vi "RT Driver VI.vi"(7 "Operation":T1, 11 "Device Reference in":T2 format="%.0x") -> (0 "Error Code":i32)   [LabVIEW 2019, in "Control Addon Engine.lvlib"]
uses:
  Control Addon Engine.lvlib
  <vilib>/NI VeriStand/Custom Device API/Custom Device Item Ref.ctl
  <vilib>/NI VeriStand/Custom Device API/Model Interface Driver VI Operation.ctl
  Types/RT Driver State Variables.ctl
  Types/RT Configuration.ctl
  Addon Shared/Types/Gain Schedule.ctl
  Addon Shared/Types/Compiled Settings.ctl
  Addon Shared/Types/Compiled PID Settings.ctl
  <vilib>/NI VeriStand/Custom Device API/Block Data Reference.ctl
  <vilib>/NI VeriStand/Custom Device API/Data Reference.ctl
  Addon Shared/Types/Compiled Industrial Settings.ctl
  Addon Shared/Types/Compiled Industrial Parameters.ctl
  <vilib>/NI/NIVS Inline Async API/_VS Inline Async API/VS Inline Async API/VS Inline Async API.lvclass
  <vilib>/NI/NIVS Inline Async API/_VS Inline Async API/VS Inline Async API/Types/Error Handling Settings.ctl
  <vilib>/NI VeriStand/Custom Device API/NI VeriStand - Get Channel Values by Block Data Reference.vi
  <vilib>/addons/control/pid/pid.llb/PID Advanced (DBL Array).vi
  <vilib>/NI VeriStand/Custom Device API/NI VeriStand - Set Channel Values by Block Data Reference.vi
  SubVIs/Get PID Gains from Schedule.vi
  SubVIs/Digital Debounce Filter.vi
  <vilib>/addons/control/pid/pid.llb/PID Parameter Manager (DBL Array).vi
  <vilib>/addons/control/pid/pid.llb/PID Derivative Action Buffered (DBL Array).vi
  <vilib>/addons/control/pid/pid.llb/PID Get Advanced Error (DBL Array).vi
  <vilib>/addons/control/pid/pid.llb/PID Integral Action Buffered (DBL Array).vi
  <vilib>/addons/control/pid/pid.llb/PID Resize 1D Array.vi
  <vilib>/addons/control/pid/pid.llb/PID Get Advanced Error (DBL).vi
  <vilib>/Utility/SystemLogging/Write to System Log.vi
  <vilib>/NI VeriStand/Custom Device API/Global Data Refs.vi
  <vilib>/addons/control/pid/pid.llb/PID Gain Schedule.vi
  <vilib>/addons/control/pid/pid.llb/PID Gain Schedule (DBL).vi
  <vilib>/addons/control/pid/pid.llb/PID Output Rate Limiter.vi
  <vilib>/addons/control/pid/pid.llb/PID Output Rate Limiter (DBL Array).vi
  Addon Shared/Control Addon Shared.lvlib
  <vilib>/NI VeriStand/Custom Device API/Custom Device API.lvlib
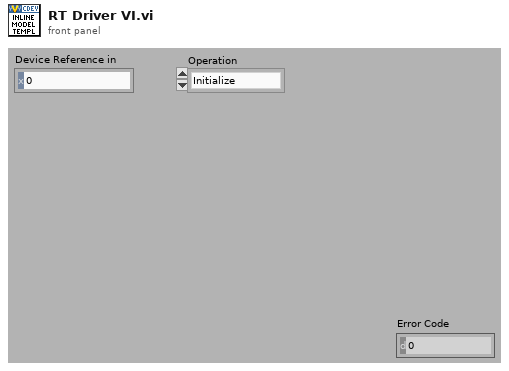
[diagram p1: front panel]
types:
  T1 = typedef "Custom Device API.lvlib/Model Interface Driver VI Operation.ctl" = enum16{"Initialize", "Start", "Execute Model", "Close"}
  T2 = typedef "Custom Device API.lvlib/Custom Device Item Ref.ctl" = u64
  T3 = typedef "Control Addon Engine.lvlib/RT Driver State Variables.ctl" = cluster{"Config":T4, "Init":bool, "Async":refnum<class "VS Inline Async API.lvclass">}
  T4 = typedef "Control Addon Engine.lvlib/RT Configuration.ctl" = cluster{"Parameter Refs":refnum<data-value>[], "Config":T5}
  T5 = typedef "Control Addon Shared.lvlib/Compiled Settings.ctl" = cluster{"PID Settings":T6, "Name":string, "Industrial Settings":T10}
  T6 = typedef "Control Addon Shared.lvlib/Compiled PID Settings.ctl" = cluster{"Gain Schedule":T7[], "Enable Live Updates":bool[], "output range":cluster{"output high":dbl, "output low":dbl}[], "setpoint range":cluster{"setpoint high":dbl, "setpoint low":dbl}[], "Write Refs":T8[], "Write Data":dbl[], "Read Refs":T8[], "Read Data":dbl[], "Control Loop Names":string[], "Enable Gain Scheduling":bool[], "Output Rate Limiter":dbl[], "dt":dbl, "setpoint high limit":dbl[], "setpoint low limit":dbl[], "output high limit":dbl[], "output low limit":dbl[]}
  T7 = typedef "Control Addon Shared.lvlib/Gain Schedule.ctl" = cluster{"Gain Schedule":cluster{"PID gains":cluster{"proportional gain (Kc)":dbl, "integral time (Ti, min)":dbl, "derivative time (Td, min)":dbl}, "max value":dbl}[]}
  T8 = typedef "Custom Device API.lvlib/Block Data Reference.ctl" = cluster{"Data Reference":T9, "Offset":u64, "Length":u64}
  T9 = typedef "Custom Device API.lvlib/Data Reference.ctl" = i32
  T10 = typedef "Control Addon Shared.lvlib/Compiled Industrial Settings.ctl" = cluster{"output range":cluster{"output high":dbl, "output low":dbl}[], "setpoint range":cluster{"setpoint high":dbl, "setpoint low":dbl}[], "Write Refs":T8[], "Write Data":dbl[], "Read Refs":T8[], "Read Data":dbl[], "Control Loop Names":string[], "Parameters":T11[], "Previous States":bool[], "Previous Counts":u64[]}
  T11 = typedef "Control Addon Shared.lvlib/Compiled Industrial Parameters.ctl" = cluster{"Enable Hysteresis":bool, "Hysteresis":dbl, "Minimum Switching":u64}
  T12 = typedef "VS Inline Async API.lvlib/VS Inline Async API.lvclass/Error Handling Settings.ctl" = cluster{"Write to SystemLog (F)":bool}
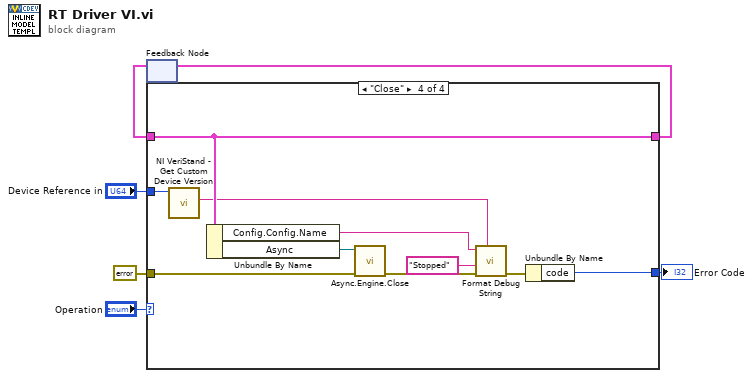
[diagram p0: block diagram]
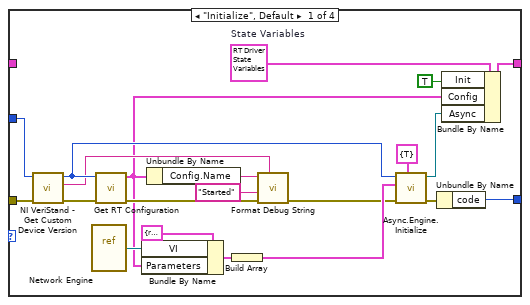
[diagram p2: hidden frame]
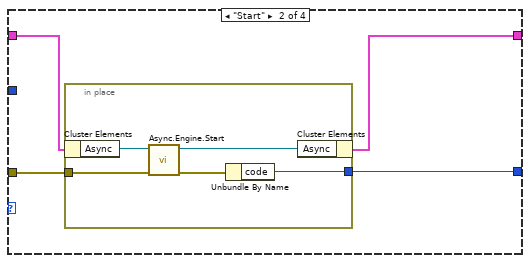
[diagram p3: hidden frame]
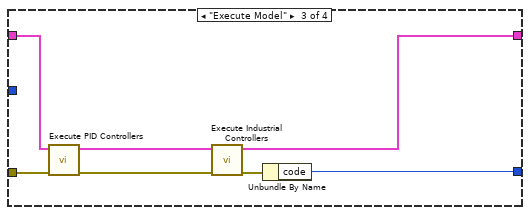
[diagram p4: hidden frame]
diagram:
  n1 = feedback #1() -> (w5:T3)  [unwired: 1 out]
  n2 = case shown="\"Close\"" "Operation" {
    tunnel: [w25 w28 w39 w53] -> w1
    tunnel: w5 -> [_ w29 w42 w53]
    tunnel: "Device Reference in" -> [w17 _ _ w48]
    tunnel: [w27 w31 w40 w52] -> w3
    tunnel: errorcluster {"status"=FALSE, "code"=0, "source"=""} ("error in (no error)") -> [w15 w30 w43 w51]
    frame "Initialize", Default {
      w23 = T3 {"Config"={"Parameter Refs"=[], "Config"={"PID Settings"={"Gain Schedule"=[], "Enable Live Updates"=[], "output range"=[], "setpoint range"=[], "Write Refs"=[], "Write Data"=[], "Read Refs"=[], "Read Data"=[], "Control Loop Names"=[], "Enable Gain Scheduling"=[], "Output Rate Limiter"=[], "dt"=0.0, "setpoint high limit"=[], "setpoint low limit"=[], "output high limit"=[], "output low limit"=[]}, "Name"="", "Industrial Settings"={"output range"=[], "setpoint range"=[], "Write Refs"=[], "Write Data"=[], "Read Refs"=[], "Read Data"=[], "Control Loop Names"=[], "Parameters"=[], "Previous States"=[], "Previous Counts"=[]}}}, "Init"=FALSE, "Async"=refnum}  # State Variables
      n3 = call <vilib>:"NI VeriStand - Get Custom Device Version.vi"("error in (no error)"=w15, "Device Ref in"=w17) -> ("error out"=w16:errorcluster, "Value"=w10:string, "Device Ref out"=w11:T2)  [unwired: 7 in]
      n4 = vi-ref "Network Engine.vi"() -> (w21:refnum<vi>)
      n5 = call "Get RT Configuration.vi"("error in (no error)"=w16, "Device Reference in"=w11) -> ("error out"=w13:errorcluster, "RT Config"=w8:T4)  [unwired: 8 in]
      n6 = Bundle By Name(cluster=cluster{"VI":refnum<vi>, "Parameters":variant} {"VI"=refnum, "Parameters"=variant} ("Process"), "VI"=w21, "Parameters"=w8) -> (w20:cluster{"VI":refnum<vi>, "Parameters":variant})
      n7 = Unbundle By Name(w8) -> ("Config.Name"=w7:string)
      n8 = Build Array(w20) -> (w19:cluster{"VI":refnum<vi>, "Parameters":variant}[])
      n9 = call "Format Debug String.vi"("Version"=w10, "error in (no error)"=w13, "State"="Started", "Name"=w7) -> ("error out"=w12:errorcluster)  [unwired: 7 in]
      n10 = call <vilib>:"Async.Engine.Initialize.vi"("Error Log Settings"=T12 {"Write to SystemLog (F)"=TRUE}, "error in (no error)"=w12, "Processes"=w19, "Custom Device Ref"=w11) -> ("error out"=w26:errorcluster, "Async"=w18:refnum<class "VS Inline Async API.lvclass">)  [unwired: 6 in]
      n11 = Unbundle By Name(w26) -> ("code"=w27:i32)
      n12 = Bundle By Name(cluster=w23, "Init"=TRUE, "Config"=w8, "Async"=w18) -> (w25:T3)
    }
    frame "Start" {
      n13 = in-place {
        in-place-border: [w36] -> w31
        in-place-border: w30 -> [w35]
        n14 = in-place-cluster #2(w29) -> ("Async"=w33:refnum<class "VS Inline Async API.lvclass">)
        n15 = call <vilib>:"Async.Engine.Start.vi"("error in (no error)"=w35, "VS Inline Async API in"=w33) -> ("error out"=w34:errorcluster, "VS Inline Async API out"=w32:refnum<class "VS Inline Async API.lvclass">)  [unwired: 8 in]
        n16 = Unbundle By Name(w34) -> ("code"=w36:i32)
        n17 = in-place-cluster #2("Async"=w32) -> (w28:T3)
      }
    }
    frame "Execute Model" {
      n18 = call "Execute PID Controllers.vi"("error in (no error)"=w43, "State Variables in"=w42) -> ("error out"=w38:errorcluster, "State Variables out"=w41:T3)  [unwired: 8 in]
      n19 = call "Execute Industrial Controllers.vi"("error in (no error)"=w38, "State Variables in"=w41) -> ("error out"=w37:errorcluster, "State Variables out"=w39:T3)  [unwired: 8 in]
      n20 = Unbundle By Name(w37) -> ("code"=w40:i32)
    }
    frame "Close" {
      n21 = call <vilib>:"NI VeriStand - Get Custom Device Version.vi"("Device Ref in"=w48) -> ("Value"=w47:string)  [unwired: 8 in, 2 out]
      n22 = Unbundle By Name(w53) -> ("Config.Config.Name"=w46:string, "Async"=w50:refnum<class "VS Inline Async API.lvclass">)
      n23 = call <vilib>:"Async.Engine.Close.vi"("error in (no error)"=w51, "Async in"=w50) -> ("error out"=w45:errorcluster)  [unwired: 8 in, 1 out]
      n24 = call "Format Debug String.vi"("Version"=w47, "error in (no error)"=w45, "State"="Stopped", "Name"=w46) -> ("error out"=w44:errorcluster)  [unwired: 7 in]
      n25 = Unbundle By Name(w44) -> ("code"=w52:i32)
    }
  }
  "Error Code" <- w3
  n26 = feedback-in #1(w1) -> ()
